vi "Prepare Control.vi"(7 "VolatusAPI":refnum<class "VolatusAPI.lvclass">, 8 "error in (no error)":errorcluster, 11 "ValveControl in":refnum<class "ValveControl.lvclass">) -> (0 "error out":errorcluster, 3 "ValveControl out":refnum<class "ValveControl.lvclass">)   [LabVIEW 2020, in "VolatusControl.lvlib" / "ValveControl.lvclass"]
uses:
  ValveControl.lvclass
  ValveControl.lvclass/ValveControl.ctl
  Volatus/VolatusAPI/VolatusAPI.lvclass
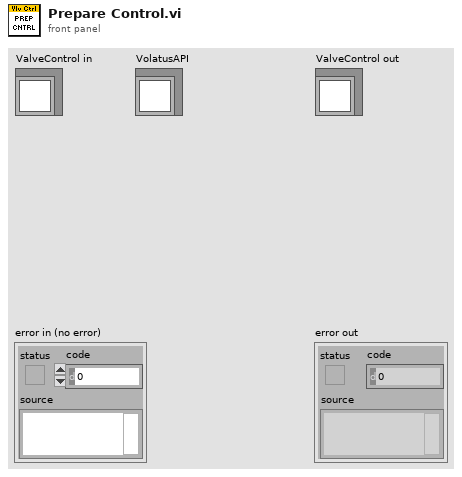
[diagram p1: front panel]
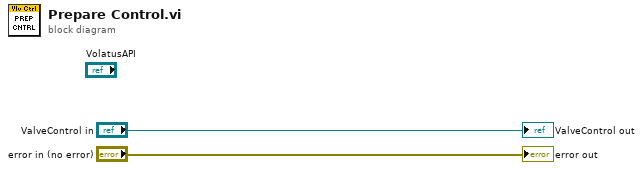
[diagram p0: block diagram]
diagram:
  "error out" <- "error in (no error)"
  "ValveControl out" <- "ValveControl in"
